vi "EditMoves.vi"() -> ()   [LabVIEW 2018]
uses:
  Drive Auton.ctl
panel:
  in  "Auton Name":string
  in  "Cancel":bool
  in  "Team Number":i32=4810
  in  "Send":bool
  in  "Save":bool
  in  "Array":T1[](array[typedef])
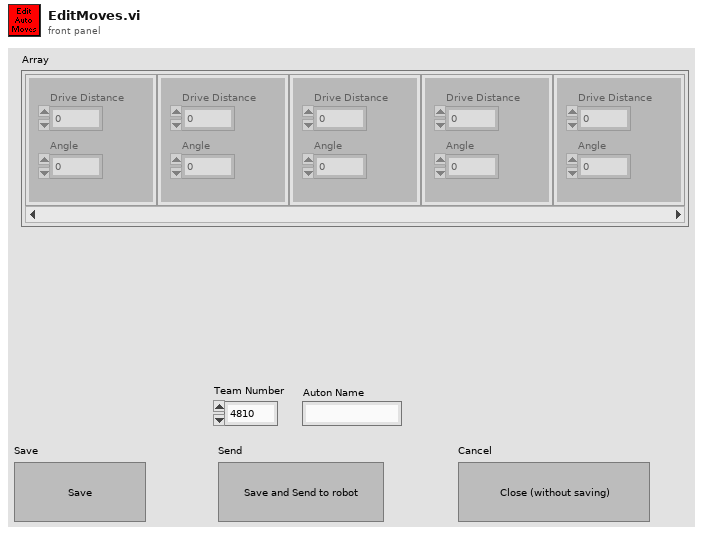
[diagram p1: front panel]
types:
  T1 = typedef "Drive Auton.ctl" = cluster{"Drive Distance":dbl, "Angle":dbl}
  T2 = enum16{"Init", "Save locally", "Update Cache", "Send to Bot", "Waiting"}
  T3 = enum16{"open", "replace", "create", "open or create", "replace or create", "replace or create with confirmation"}
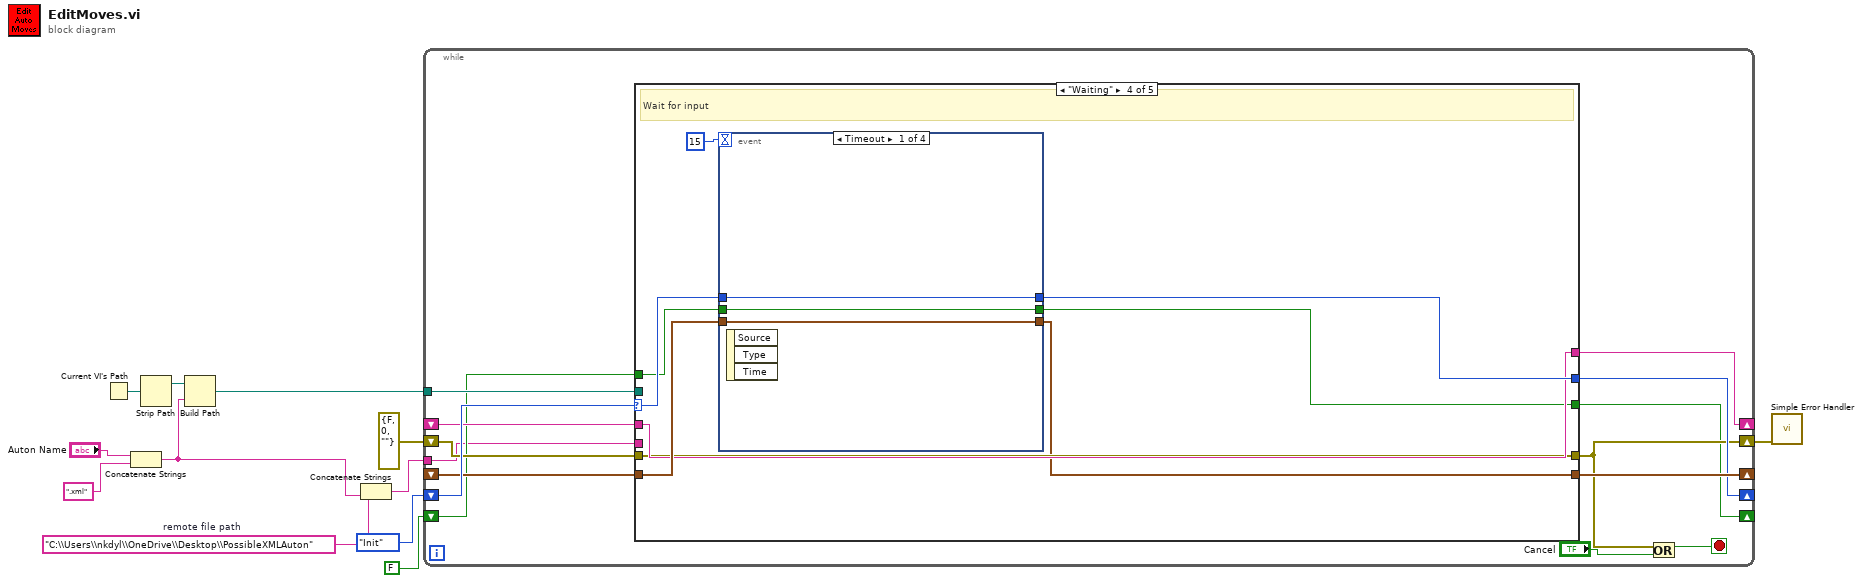
[diagram p0: block diagram]
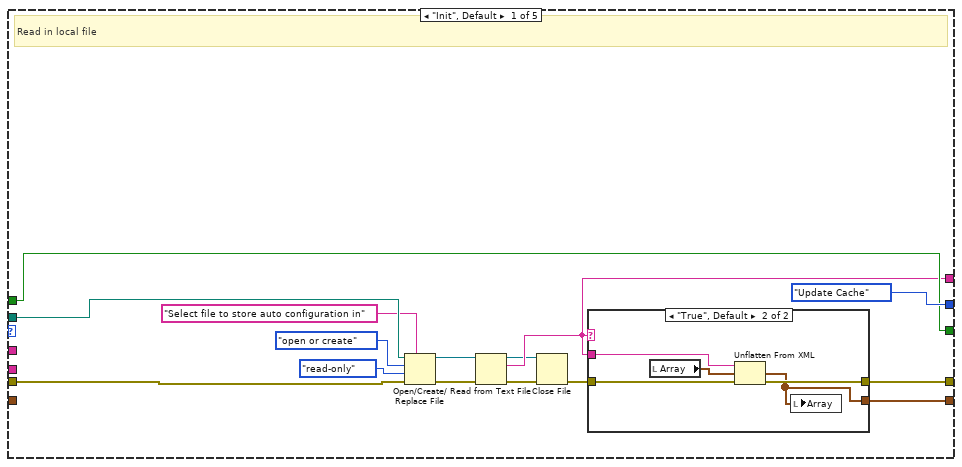
[diagram p2: hidden frame]
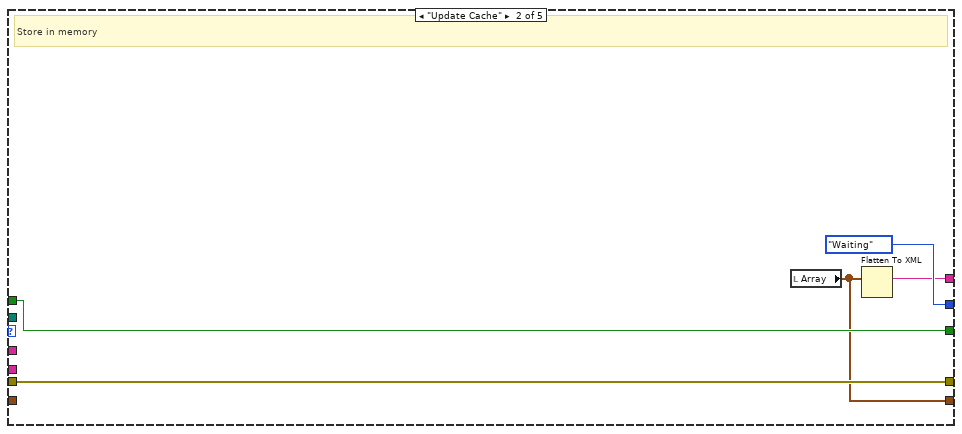
[diagram p4: hidden frame]
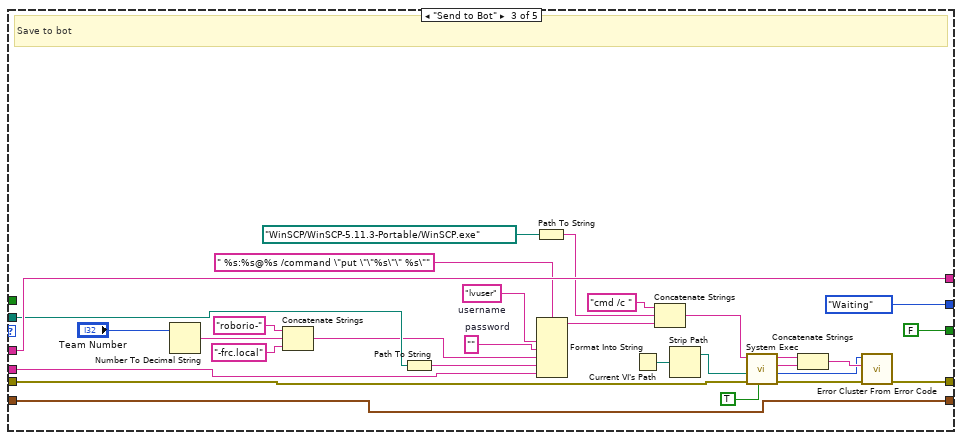
[diagram p5: hidden frame]
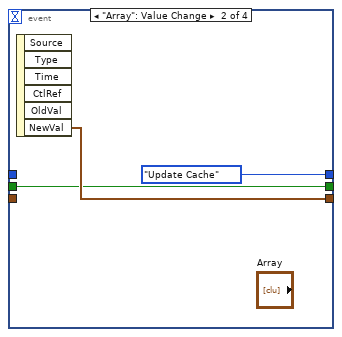
[diagram p6: hidden frame]
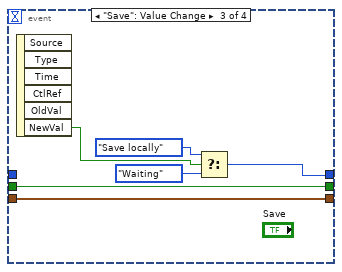
[diagram p7: hidden frame]
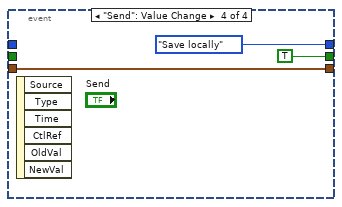
[diagram p8: hidden frame]
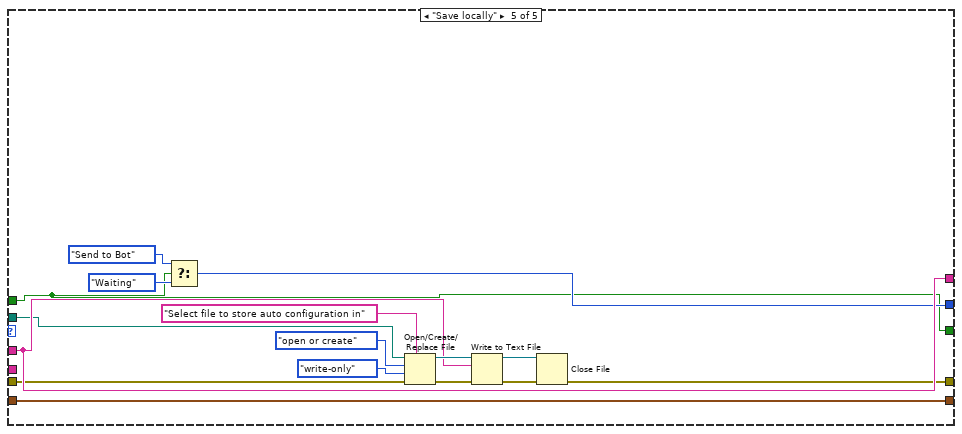
[diagram p9: hidden frame]
diagram:
  w5 = "C:\\Users\\nkdyl\\OneDrive\\Desktop\\PossibleXMLAuton"  # remote file path
  n1 = Current VI's Path() -> (path=w9:path)
  n2 = Concatenate Strings("Auton Name", ".xml") -> (w2:string)
  n3 = Strip Path(path=w9) -> (stripped path=w8:path)  [unwired: 1 out]
  n4 = Build Path(base path=w8, name or relative path=w2) -> (appended path=w7:path)
  n5 = Concatenate Strings(w5, w2) -> (w1:string)
  n6 = while {
    shift-right: [w24] -> _
    shift-left: T2."Init" -> [w26]
    shift-right: [w25] -> _
    shift-left: _ -> [w23]
    shift-right: [w22] -> _
    shift-left: _ -> [w18]
    shift-right: [w21] -> w10
    shift-left: errorcluster {"status"=FALSE, "code"=0, "source"=""} ("error out") -> [w19]
    tunnel: w7 -> [w20]
    shift-right: [w16] -> _
    shift-left: FALSE -> [w17]
    tunnel: w1 -> [w15]
    stop <- w14 stop-if-true
    n7 = case shown="\"Waiting\"" w26 {
      selector: w26 -> [_ _ _ w89 _]
      tunnel: [w27 w48 w82 w83 w122] -> w25
      tunnel: [T2."Update Cache" T2."Waiting" T2."Waiting" w91 w111] -> w24
      tunnel: w23 -> [_ _ w82 w90 w122]
      tunnel: [w35 w49 w81 w87 w114] -> w22
      tunnel: [w38 w50 w73 w86 w109] -> w21
      tunnel: w20 -> [w37 _ w77 _ w107]
      tunnel: w19 -> [w36 w50 w76 w86 w108]
      tunnel: w18 -> [_ _ w81 w87 w114]
      tunnel: w17 -> [w40 w51 _ w84 w110]
      tunnel: [w40 w51 FALSE w85 w110] -> w16
      tunnel: w15 -> [_ _ w62 _ _]
      frame "Init", Default {
        # "Read in local file"
        n8 = Open/Create/Replace File(file path (use dialog)=w37, error in=w36, prompt="Select file to store auto configuration in", operation (0:open)=T3."open or create", access (0:read/write)=enum16{"read/write", "read-only", "write-only"}."read-only") -> (refnum out=w31:refnum<file>, error out=w30:errorcluster)  [unwired: 1 in, 1 out]
        n9 = Read from Text File(file (use dialog)=w31, error in=w30) -> (refnum out=w28:refnum<file>, text=w35:string, error out=w29:errorcluster)  [unwired: 2 in, 1 out]
        n10 = Close File(refnum=w28, error in=w29) -> (error out=w39:errorcluster)  [unwired: 1 out]
        n11 = case shown="\"True\", Default" w35 {
          tunnel: w35 -> [_ w47]
          tunnel: w39 -> [w42 w45]
          tunnel: [w42 w44] -> w38
          tunnel: [_ w43] -> w27
          frame "" {
          }
          frame "True", Default {
            n12 = local read "Array"() -> (w46:T1[])
            n13 = Unflatten From XML(xml string=w47, type=w46, error in (no error)=w45) -> (value=w43:T1[], error out=w44:errorcluster)
            n14 = local write "Array"(w43) -> ()
          }
        }
      }
      frame "Update Cache" {
        # "Store in memory"
        n15 = local read "Array"() -> (w48:T1[])
        n16 = Flatten To XML(anything=w48) -> (xml string=w49:string)
      }
      frame "Send to Bot" {
        w66 = ""  # password
        w67 = "lvuser"  # username
        # "Save to bot"
        n17 = Number To Decimal String(number="Team Number") -> (decimal integer string=w53:string)  [unwired: 1 in]
        n18 = Concatenate Strings("roborio-" ("string"), w53, "-frc.local" ("string")) -> (w65:string)
        n19 = Path To String(path=w77) -> (string=w64:string)
        n20 = Path To String(path=path "WinSCP/WinSCP-5.11.3-Portable/WinSCP.exe") -> (string=w57:string)
        n21 = Format Into String(format string=" %s:%s@%s /command \"put \"\"%s\"\" %s\"", w67, w66, w65, w64, w62) -> (resulting string=w63:string)  [unwired: 2 in, 1 out]
        n22 = Current VI's Path() -> (path=w78:path)
        n23 = Concatenate Strings("cmd /c " ("string"), w57, w63) -> (w59:string)
        n24 = Strip Path(path=w78) -> (stripped path=w68:path)  [unwired: 1 out]
        n25 = call <vilib>:"System Exec.vi"("run minimized? (F)"=TRUE, "error in (no error)"=w76, "working directory"=w68, "command line"=w59) -> ("error out"=w74:errorcluster, "return code"=w69:i32, "standard error"=w70:string, "standard output"=w71:string)  [unwired: 4 in]
        n26 = Concatenate Strings(w71, w70) -> (w72:string)
        n27 = call <vilib>:"Error Cluster From Error Code.vi"("error in (no error)"=w74, "error message (\"\")"=w72, "error code (0)"=w69) -> ("error out"=w73:errorcluster)  [unwired: 6 in]
      }
      frame "Waiting" {
        # "Wait for input"
        n28 = event shown="[0] Timeout" {
          selector: _ -> [_ _ _ _]
          dyn-events: _ -> [_ _ _ _]
          timeout: 15 -> [_ _ _ _]
          tunnel: [w92 w97 w98 w104] -> w83
          tunnel: [w94 T2."Update Cache" w102 T2."Save locally"] -> w91
          tunnel: w90 -> [w92 _ w98 w104]
          tunnel: w89 -> [w94 _ _ _]
          tunnel: [w93 w95 w99 TRUE] -> w85
          tunnel: w84 -> [w93 w95 w99 _]
          event Timeout {
            n29 = event-data() -> ()  [unwired: 1 in, 3 out]
          }
          event "Array": Value Change {
            n30 = event-data() -> ("NewVal"=w97:T1[])  [unwired: 1 in, 5 out]
          }
          event "Save": Value Change {
            n31 = event-data() -> ("NewVal"=w103:bool)  [unwired: 1 in, 5 out]
            n32 = Select(t=T2."Save locally", s=w103, f=T2."Waiting") -> (s? t:f=w102:T2)
          }
          event "Send": Value Change {
            n33 = event-data() -> ()  [unwired: 1 in, 6 out]
          }
        }
      }
      frame "Save locally" {
        n34 = Select(t=T2."Send to Bot", s=w110, f=T2."Waiting") -> (s? t:f=w111:T2)
        n35 = Open/Create/Replace File(file path (use dialog)=w107, error in=w108, prompt="Select file to store auto configuration in", operation (0:open)=T3."open or create", access (0:read/write)=enum16{"read/write", "read-only", "write-only"}."write-only") -> (refnum out=w118:refnum<file>, error out=w117:errorcluster)  [unwired: 1 in, 1 out]
        n36 = Write to Text File(file (use dialog)=w118, text=w114, error in=w117) -> (refnum out=w115:refnum<file>, error out=w116:errorcluster)  [unwired: 1 in, 1 out]
        n37 = Close File(refnum=w115, error in=w116) -> (error out=w109:errorcluster)  [unwired: 1 out]
      }
    }
    n38 = Or(x=w21, y="Cancel") -> (x .or. y?=w14:bool)
  }
  n39 = call <vilib>:"Simple Error Handler.vi"("error in (no error)"=w10) -> ()  [unwired: 4 in, 5 out]
